vi "TDMS.CheckFileProperties.vi"(8 "error in (no error)":errorcluster, 11 "Data":path) -> (0 "error out":errorcluster, 3 "Found All":bool)   [LabVIEW 2014, in "NIAnalysis.lvlib"]
uses:
  NIAnalysis.lvlib
  Constants.vi
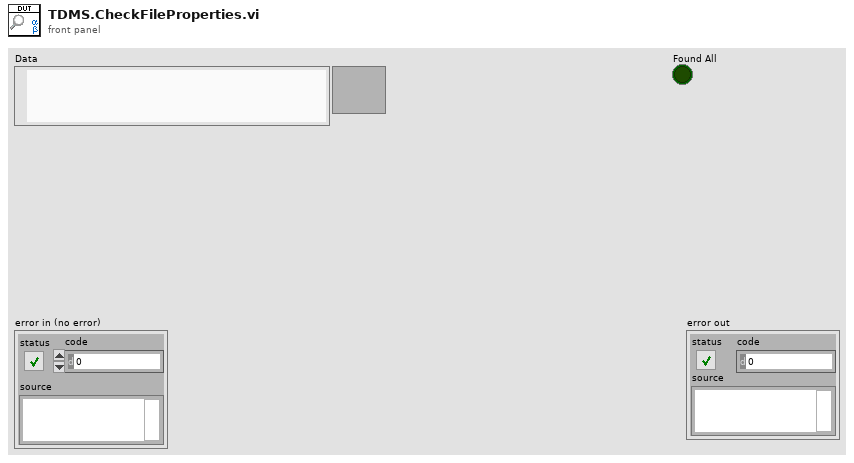
[diagram p1: front panel]
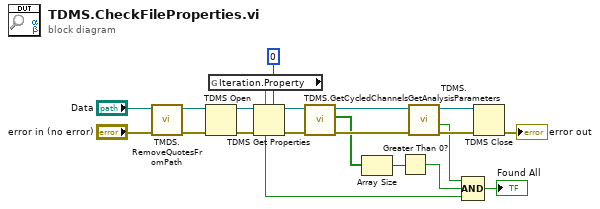
[diagram p0: block diagram]
diagram:
  n1 = call "TMDS.RemoveQuotesFromPath.vi"("error in (no error)"="error in (no error)", "Data"="Data") -> ("error out"=w3:errorcluster, "Path"=w2:path)  [unwired: 8 in]
  n2 = TDMS Open(8:w3, 11:w2) -> (0:w18:errorcluster, 3:w19:refnum<k34>)  [unwired: 5 in]
  n3 = global read "Constants.vi" "Iteration.Property"() -> (w20:string)
  n4 = TDMS Get Properties(5:0 ("Iteration"), 7:w20, 8:w18, 11:w19) -> (0:w11:errorcluster, 3:w10:refnum<k34>, 6:w16:bool)  [unwired: 2 in, 3 out]
  n5 = call "TDMS.GetCycledChannels.vi"("error in (no error)"=w11, "TDMS Ref"=w10) -> ("error out"=w8:errorcluster, "Cycled"=w7:bool[], "TDMS Ref"=w9:refnum<k34>)  [unwired: 6 in, 1 out]
  n6 = Array Size(array=w7) -> (size(s)=w6:i32)
  n7 = Greater Than 0?(x=w6) -> (x > 0?=w5:bool)
  n8 = call "TDMS.GetAnalysisParameters.vi"("error in (no error)"=w8, "TDMS Ref"=w9) -> ("error out"=w14:errorcluster, "Found?"=w12:bool, "TDMS Ref"=w13:refnum<k34>)  [unwired: 6 in, 1 out]
  n9 = Compound Arithmetic op=AND(w12, w5, w16) -> (→"Found All":bool)
  n10 = TDMS Close(8:w14, 11:w13) -> (0:→"error out":errorcluster)  [unwired: 1 out]
